vi "Get motor RPM, current, power, torque.vi"(4 "Drive address":T4=1 items=["0", "1", "2", "3", "4", "5", "6", "7", "8", "9", "10", "11", "12", "13", "14", "15", "16", "17", "18", "19", "20", "21", "22", "23", "24", "25", "26", "27", "28", "29", "30", "31", "32", "33", "34", "35", "36", "37", "38", "39", "40", "41", "42", "43", "44", "45", "46", "47", "48", "49", "50", "51", "52", "53", "54", "55", "56", "57", "58", "59", "60", "61", "62", "63"], 5 "COM port":refnum<visa-resource-name>) -> (0 "Motor data":T3, 1 "Modbus error cluster":T1={"Checksum ok"=FALSE, "Modbus exception code"=1, "Response from correct drive"=FALSE, "Comms error"={"status"=FALSE, "code"=0, "source"=""}} {"Modbus exception code" items=["None"=0, "Invalid function request"=1, "Invalid Modbus register address"=2, "Invalid / unauthorised data value"=3, "Device failure"=4, "Request accepted, wait"=5, "Drive busy"=6, "Request rejected"=7, "Memory parity error"=8, "Gateway path unavailable"=10, "Device failed to respond"=11]}, 2 "No errors":bool)   [LabVIEW 2020]
doc: "Modbus RTU for Invertek drives. Paul Nathan 21-JUN-2022."
uses:
  ctls/Drive address.ctl
  ctls/Motor data.ctl
  ctls/Register.ctl
  ctls/Exception codes.ctl
  ctls/Modbus error cluster.ctl
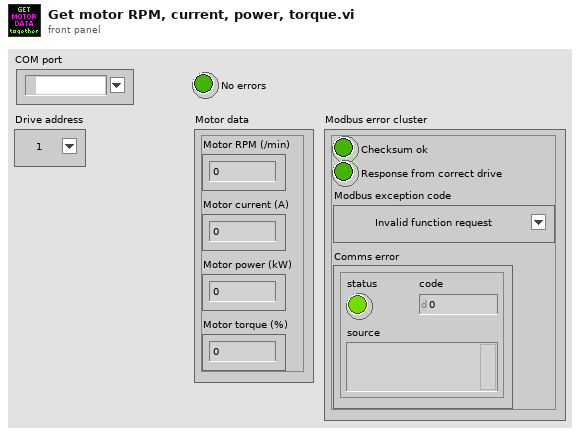
[diagram p1: front panel]
types:
  T1 = typedef "Modbus error cluster.ctl" = cluster{"Checksum ok":bool, "Modbus exception code":T2, "Response from correct drive":bool, "Comms error":errorcluster}
  T2 = typedef "Exception codes.ctl" = u8
  T3 = typedef "Motor data.ctl" = cluster{"Motor RPM (/min)":dbl, "Motor current (A)":dbl, "Motor power (kW)":dbl, "Motor torque (%)":dbl}
  T4 = typedef "Drive address.ctl" = u8
  T5 = typedef "Register.ctl" = u16
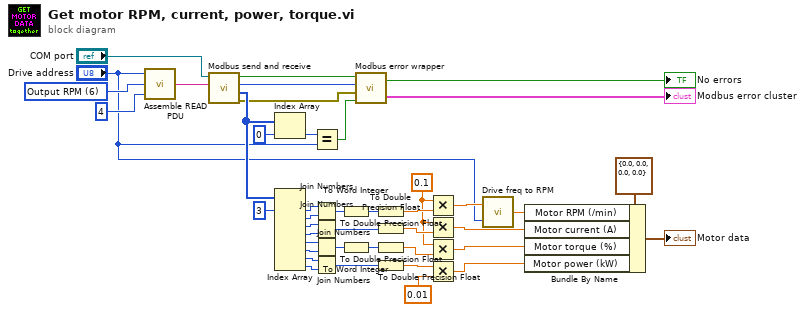
[diagram p0: block diagram]
diagram:
  w10 = T5 6 items=["Control"=0, "RPM set-point"=4, "Drive status"=5, "Output RPM"=6, "Motor current"=7, "Motor torque"=8, "Motor power"=9, "DC bus voltage"=22, "Drive power stage temperature"=23, "kWh meter"=31, "MWh meter"=32, "Running time - hours"=33, "Running time - seconds"=34, "Internal drive temperature"=38, "Motor RMS voltage"=42, "Extended drive status"=2000] ("Register")
  w20 = 0.1 ("y")
  n1 = call "Assemble READ PDU.vi"("No. of registers"=u16 4, "Register"=w10, "Drive address"="Drive address") -> ("Ser out string"=w42:string)
  n2 = call "Modbus send and receive.vi"("Modbus telegram"=w42, "COM port"="COM port") -> ("Comms error"=w3:errorcluster, "Device response"=w37:u8[], "Modbus exception code"=w2:T2, "Checksum ok"=w1:bool)  [unwired: 2 in]
  n3 = Index Array(array=w37, index=0) -> (element=w39:u8)
  n4 = Index Array(array=w37, index #1=3 ("index")) -> (element #1=w35:u8, element #2=w34:u8, element #3=w31:u8, element #4=w30:u8, element #5=w29:u8, element #6=w28:u8, element #7=w27:u8, element #8=w26:u8)  [unwired: 7 in]
  n5 = Equal?(x=w39, y="Drive address") -> (x = y?=w4:bool)
  n6 = Join Numbers(hi=w35, lo=w34) -> ((hi.lo)=w33:u16)
  n7 = Join Numbers(hi=w31, lo=w30) -> ((hi.lo)=w24:u16)
  n8 = Join Numbers(hi=w29, lo=w28) -> ((hi.lo)=w25:u16)
  n9 = Join Numbers(hi=w27, lo=w26) -> ((hi.lo)=w23:u16)
  n10 = To Word Integer(number=w33) -> (16bit integer=w32:i16)
  n11 = To Word Integer(number=w25) -> (16bit integer=w19:i16)
  n12 = call "Modbus error wrapper.vi"("Response from correct drive"=w4, "Comms error"=w3, "Modbus exception code"=w2, "Checksum ok"=w1) -> ("Modbus error cluster"=→"Modbus error cluster":T1, "No errors"=→"No errors":bool)
  n13 = To Double Precision Float(number=w32) -> (double precision float=w22:dbl)
  n14 = To Double Precision Float(number=w24) -> (double precision float=w21:dbl)
  n15 = To Double Precision Float(number=w19) -> (double precision float=w18:dbl)
  n16 = To Double Precision Float(number=w23) -> (double precision float=w17:dbl)
  n17 = Multiply(x=w20, y=w22) -> (x*y=w9:dbl)
  n18 = Multiply(x=w20, y=w21) -> (x*y=w15:dbl)
  n19 = Multiply(x=w20, y=w18) -> (x*y=w14:dbl)
  n20 = Multiply(x=w17, y=0.01) -> (x*y=w13:dbl)
  n21 = call "Drive freq to RPM.vi"("Drive address"="Drive address", "Drive output f (Hz)"=w9) -> ("Motor RPM (/min)"=w8:dbl)
  n22 = Bundle By Name(cluster=T3 {"Motor RPM (/min)"=0.0, "Motor current (A)"=0.0, "Motor power (kW)"=0.0, "Motor torque (%)"=0.0} ("Motor stats"), "Motor RPM (/min)"=w8, "Motor current (A)"=w15, "Motor torque (%)"=w14, "Motor power (kW)"=w13) -> (→"Motor data":T3)
